vi "Login-Window2.vi"(7 "PwdMgr":refnum<class "PwdMgr.lvclass">, 8 "Error in":errorcluster caption="Error in (no error)", 11 "Options":T1={"HideMain(T)"=TRUE, "RetryAllowed(T)"=TRUE, "LastUserToINI(T)"=TRUE, "Titlebar(T)"=TRUE}) -> (0 "Error out":errorcluster={"status"=TRUE, "code"=43, "source"="Operation cancelled by user."}, 1 "Valid User":bool, 3 "User Info":T2={"UserName"="", "Password"="", "Role"=enum."Admin"})   [LabVIEW 2020]
uses:
  _Typedef/User-Info.ctl
  _Typedef/User-Role.ctl
  PwdMgr/PwdMgr.lvclass
  Login-Options.ctl
  Login-UI.lvlib
panel:
  in  "UserManage":bool
  in  "Login":bool
  in  "Password":string caption="密码"
  in  "UserName":string caption="用户名"
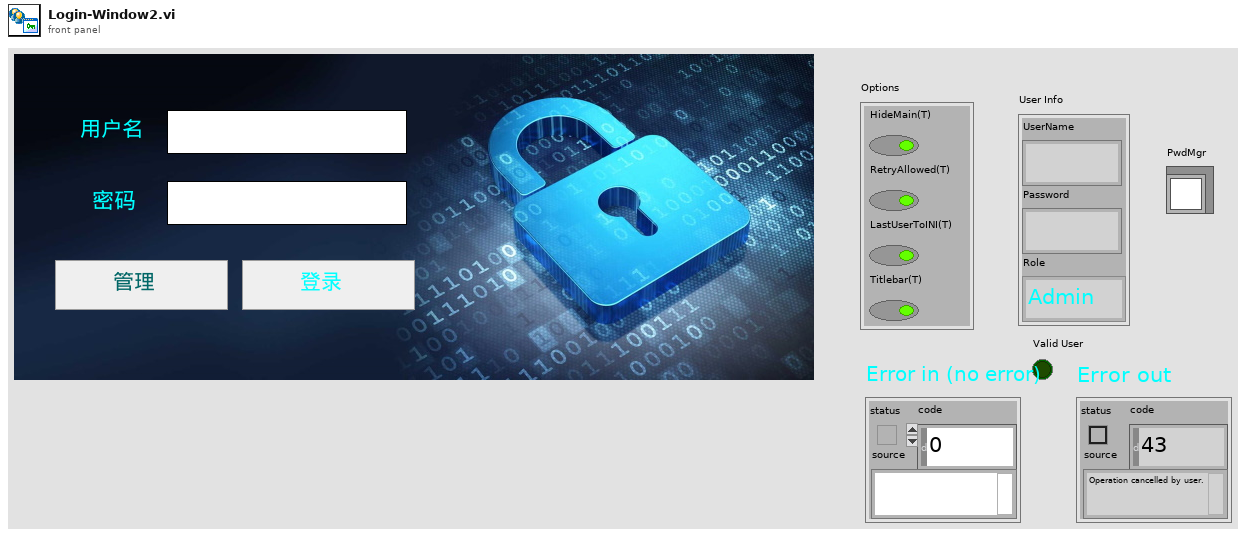
[diagram p1: front panel]
types:
  T1 = typedef "Login-UI.lvlib/Login-Options.ctl" = cluster{"HideMain(T)":bool, "RetryAllowed(T)":bool, "LastUserToINI(T)":bool, "Titlebar(T)":bool}
  T2 = typedef "Login-UI.lvlib/User-Info.ctl" = cluster{"UserName":string, "Password":string, "Role":T3}
  T3 = typedef "Login-UI.lvlib/User-Role.ctl" = enum16{"INVALID", "Operator", "Engineer", "Admin", "Anonymous"}
  T4 = cluster{"UserName":refnum<vi>, "Password ":refnum<vi>, "UserManage":refnum<vi>, "Login":refnum<vi>, "This VI":refnum<vi>, "VI Ref":refnum<vi>}
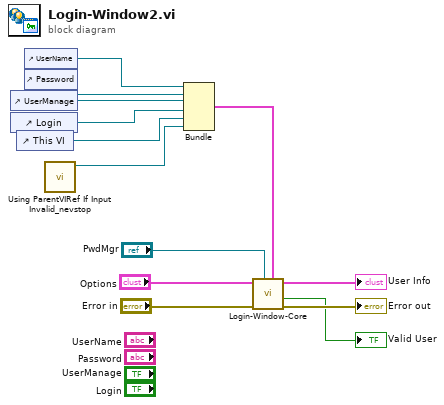
[diagram p0: block diagram]
diagram:
  n1 = control-ref of="UserManage"() -> (w5:refnum<vi>)
  n2 = control-ref of="Login"() -> (w4:refnum<vi>)
  n3 = control-ref of="This VI"() -> (w3:refnum<vi>)
  n4 = control-ref of="UserName"() -> (w7:refnum<vi>)
  n5 = control-ref of="Password"() -> (w6:refnum<vi>)
  n6 = call <userlib>:"Using ParentVIRef If Input Invalid_nevstop.vi"() -> ("VI Ref"=w1:refnum<vi>)  [unwired: 6 in, 1 out]
  n7 = Bundle("UserName"=w7, "Password"=w6, "UserManage"=w5, "Login"=w4, "This VI"=w3, "VI Ref"=w1) -> (w2:T4)  [unwired: 1 in]
  n8 = call "Login-Window-Core.vi"("Cluster"=w2, "PwdMgr"="PwdMgr", "Error in"="Error in", "Options"="Options") -> ("Error out"=→"Error out":errorcluster, "Valid User"=→"Valid User":bool, "User Info"=→"User Info":T2)  [unwired: 5 in]
